vi "edge_to_points(subVI).vi"(8 "error in (no error)":errorcluster, 11 "First Edges":T1[](array[typedef]) {"Distance (Real-World)" format="%.2f"; "Location (Real-World)"."Y" format="%.2g"; "Location (Real-World)"."X" format="%.2f"; "Noise" format="%.2f"; "Location (Pixel)"."Y" format="%.2g"; "Location (Pixel)"."X" format="%.2f"; "Strength" format="%.2f"; "Distance (Pixel)" format="%.2f"}) -> (0 "error out":errorcluster, 2 "points (real-world)":cluster{"X":sgl, "Y":sgl}[](array[cluster]), 3 "points (pixel)":cluster{"X":sgl, "Y":sgl}[](array[cluster]))   [LabVIEW 2020]
uses:
  <vilib>/vision/Measure.llb/Edge New.ctl
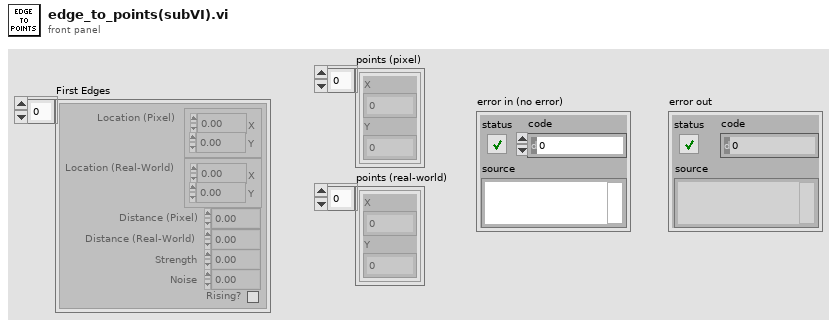
[diagram p1: front panel]
types:
  T1 = typedef "Edge New.ctl" = cluster{"Location (Pixel)":cluster{"X":sgl, "Y":sgl}, "Location (Real-World)":cluster{"X":sgl, "Y":sgl}, "Distance (Pixel)":dbl, "Distance (Real-World)":dbl, "Strength":dbl, "Noise":dbl, "Rising?":bool}
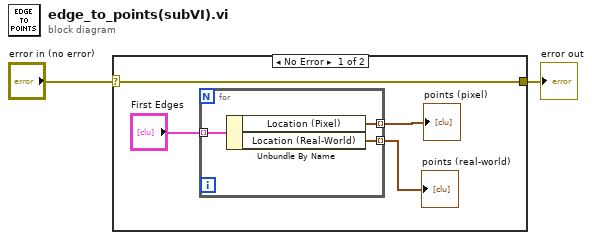
[diagram p0: block diagram]
diagram:
  n1 = case shown="No Error" "error in (no error)" {
    selector: "error in (no error)" -> [w3 w10]
    tunnel: [w3 w10] -> w1
    frame No Error {
      n2 = for {
        tunnel: "First Edges" -> [w9] mode=indexing
        tunnel: [w8] -> w5 mode=indexing
        tunnel: [w7] -> w4 mode=indexing
        n3 = Unbundle By Name(w9) -> ("Location (Pixel)"=w8:cluster{"X":sgl, "Y":sgl}, "Location (Real-World)"=w7:cluster{"X":sgl, "Y":sgl})
      }
      "points (pixel)" <- w5
      "points (real-world)" <- w4
    }
    frame Error {
    }
  }
  "error out" <- w1
